vi "DualEncoder.vi"(8 "error in (no error)":errorcluster, 11 "Reset?":bool) -> (0 "error out":errorcluster, 1 "Distance Right (in)":dbl, 2 "Distance Left (in)":dbl, 3 "Total Distance (in)":dbl)   [LabVIEW 2012]
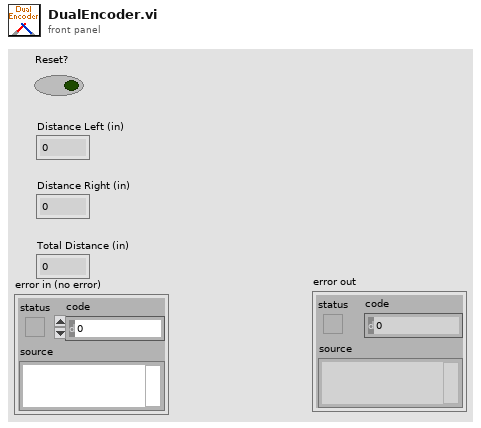
[diagram p1: front panel]
types:
  T1 = typedef "WPI_EncoderDevRef.ctl" = cluster{"DevStatus":errorcluster, "EncoderIndex":T2, "CounterIndex":T3, "DistancePerCount":dbl, "Decoding Type":T4}
  T2 = typedef "FPGA_EncoderIdx.ctl" = enum8{"Enc 0", "Enc 1", "Enc 2", "Enc 3", "Invalid"}
  T3 = typedef "FPGA_CounterCtrSystemIndex.ctl" = enum8{"Ctr 0", "Ctr 1", "Ctr 2", "Ctr 3", "Ctr 4", "Ctr 5", "Ctr 6", "Ctr 7", "Invalid"}
  T4 = typedef "WPI_EncoderType.ctl" = enum16{"1x", "2x", "4x"}
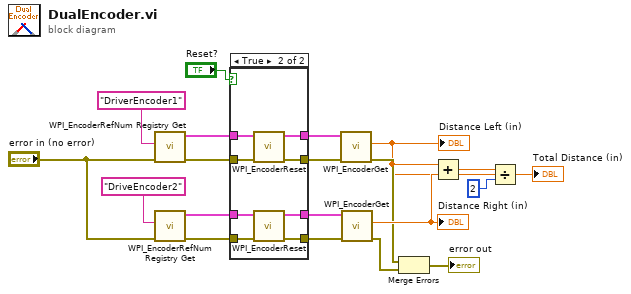
[diagram p0: block diagram]
diagram:
  n1 = call <vilib>:"WPI_EncoderRefNum Registry Get.vi"("error in (no error)"="error in (no error)", "refnum name"="DriverEncoder1") -> ("error out"=w13:errorcluster, "EncoderDevRef"=w14:T1)  [unwired: 8 in]
  n2 = call <vilib>:"WPI_EncoderRefNum Registry Get.vi"("error in (no error)"="error in (no error)", "refnum name"="DriveEncoder2") -> ("error out"=w15:errorcluster, "EncoderDevRef"=w16:T1)  [unwired: 8 in]
  n3 = case shown="True" "Reset?" {
    tunnel: w16 -> [w21 w31]
    tunnel: w15 -> [w20 w30]
    tunnel: w14 -> [w23 w29]
    tunnel: w13 -> [w22 w28]
    tunnel: [w23 w27] -> w11
    tunnel: [w22 w26] -> w10
    tunnel: [w21 w25] -> w9
    tunnel: [w20 w24] -> w8
    frame False {
    }
    frame True {
      n4 = call <vilib>:"WPI_EncoderReset.vi"("error in (no error)"=w28, "EncoderDevRef"=w29) -> ("error out"=w26:errorcluster, "EncoderDevRef"=w27:T1)  [unwired: 8 in]
      n5 = call <vilib>:"WPI_EncoderReset.vi"("error in (no error)"=w30, "EncoderDevRef"=w31) -> ("error out"=w24:errorcluster, "EncoderDevRef"=w25:T1)  [unwired: 8 in]
    }
  }
  n6 = call <vilib>:"WPI_EncoderGet.vi"("error in (no error)"=w10, "EncoderDevRef"=w11) -> ("error out"=w3:errorcluster, "Distance"=w1:dbl)  [unwired: 4 in, 4 out]
  "Distance Left (in)" <- w1
  "Total Distance (in)" <- w1
  n7 = call <vilib>:"WPI_EncoderGet.vi"("error in (no error)"=w8, "EncoderDevRef"=w9) -> ("error out"=w2:errorcluster, "Distance"=w5:dbl)  [unwired: 4 in, 4 out]
  "Distance Right (in)" <- w5
  n8 = Merge Errors(w3, w2) -> (→"error out":errorcluster)
  n9 = Add(x=w1, y=w5) -> (x+y=w6:dbl)
  n10 = Divide(x=w6, y=2) -> ()  [unwired: 1 out]
